vi "LVClass_WavefrontCorrectorSet Set Parameter Bool Value.vi"(0 "WavefrontCorrectorSet in":refnum<class "WavefrontCorrectorSet.lvclass">, 5 "parameter_name":string, 7 "Value":bool, 11 "error in (no error)":errorcluster) -> (4 "WavefrontCorrectorSet out":refnum<class "WavefrontCorrectorSet.lvclass">, 15 "error out":errorcluster)   [LabVIEW 2020, in "WavefrontCorrectorSet.lvclass"]
doc: "WavefrontCorrector parameter default value getter for parameter of type\nboolean.\n\n--------------------------------------------------------------------------------\n\n<B>wavefrontcorrector_setIn </B> : WavefrontCorrectorSet object.\n<B>wavefrontcorrector_setOut </B> : WavefrontCorrectorSet object.\n<B>parameter_name </B> : Parameter name.\n<B>default_value </B> : Parameter default value.\n<B>ErrorIn </B> : Error\n<B>ErrorOut </B> : Error\n\n--------------------------------------------------------------------------------"
uses:
  WavefrontCorrectorSet.lvclass
  WavefrontCorrectorSet.lvclass/WavefrontCorrectorSet.ctl
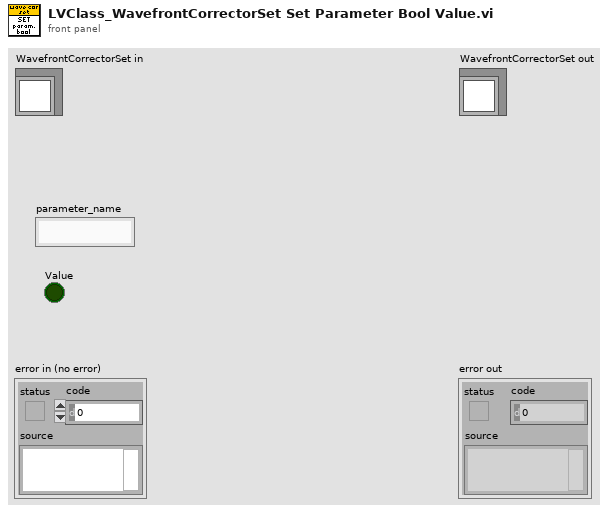
[diagram p1: front panel]
types:
  T1 = typedef "ClassID.ctl" = i64
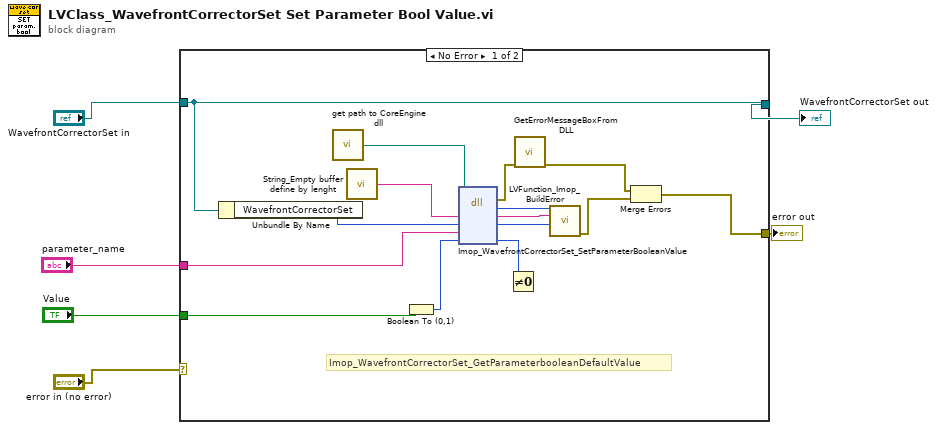
[diagram p0: block diagram]
diagram:
  n1 = case shown="No Error" "error in (no error)" {
    selector: "error in (no error)" -> [_ w22]
    tunnel: "WavefrontCorrectorSet in" -> [w14 w23]
    tunnel: [w14 w23] -> w4
    tunnel: [w12 w22] -> w3
    tunnel: "parameter_name" -> [w9 _]
    tunnel: "Value" -> [w8 _]
    frame No Error {
      # "Imop_WavefrontCorrectorSet_GetParameterbooleanDefaultValue"
      n2 = Unbundle By Name(w14) -> ("WavefrontCorrectorSet"=w13:T1)
      n3 = call "get path to CoreEngine dll.vi"() -> ("path to wavekit library"=w18:path)  [unwired: 14 in, 1 out]
      n4 = call "String_Empty buffer define by lenght.vi"() -> ("Empty buffer"=w19:string)  [unwired: 1 in]
      n5 = Boolean To (0,1)(Boolean=w8) -> (0, 1=w16:i16)
      n6 = dll-call lib="D:/soft/HASO_v3/SVN_trunk/ImOpCoreEngine4_LV2011/DLLs/c_interface_vc100.dll" fn="Imop_WavefrontCorrectorSet_SetParameterBooleanValue"(path in=w18, "message"=w19, "objet"=w13, "parameter_name"=w9, "Value"=w16) -> (error out=w17:errorcluster, "return type"=w21:i32, "message"=w20:string, "objet"=w7:i64, "Value"=w15:u8)  [unwired: 3 in, 1 out]
      n7 = Not Equal To 0?(x=w15) -> ()  [unwired: 1 out]
      n8 = call "GetErrorMessageBoxFromDLL.vi"("error IN"=w17) -> ("error OUT"=w11:errorcluster)  [unwired: 10 in]
      n9 = call "LVFunction_Imop_BuildError.vi"("code"=w21, "String to Prepend to source (\"\")"=w20, "Adresse"=w7) -> ("error out"=w10:errorcluster)  [unwired: 12 in]
      n10 = Merge Errors(w11, w10) -> (w12:errorcluster)
    }
    frame Error {
    }
  }
  "error out" <- w3
  "WavefrontCorrectorSet out" <- w4
